vi "Test Process Wait For Lifecycle State After Clearing Throws Error.vi"(8 "error in (no error)":errorcluster, 11 "Process Test In":refnum<class "Process Dev Test.lvclass">) -> (0 "error out":errorcluster, 3 "Process Test Out":refnum<class "Process Dev Test.lvclass">)   [LabVIEW 2020, in "Process Dev Test.lvclass"]
uses:
  Process Dev Test.lvclass
  C:/Program Files (x86)/National Instruments/LabVIEW 2020/vi.lib/Astemes/LUnit/Test Case.lvclass
  source/Framework/Process/Public/Lifecycle/Lifecycle State.ctl
  <vilib>/Astemes/LUnit/Test Case.lvclass/Test Case.ctl
  <vilib>/Astemes/LUnit/LUnit Assertion Result.lvclass/LUnit Assertion Result.ctl
  <vilib>/Astemes/LUnit/LUnit Test Case Result.lvclass/LUnit Test Case Result.ctl
  <vilib>/Astemes/LUnit/LUnit Method Result.lvclass/LUnit Method Result.ctl
  <vilib>/Astemes/LUnit/Palette/Fail.vi
  <vilib>/Astemes/LUnit/Palette/Pass.vi
  <vilib>/Astemes/LUnit/Set Assertion Type.vi
  <vilib>/Astemes/LUnit/Add test result.vi
  <vilib>/Astemes/LUnit/LUnit Write Passed.vi
  <vilib>/Astemes/LUnit/LUnit Write Message.vi
  <vilib>/Astemes/LUnit/LUnit Write Description.vi
  <vilib>/Astemes/LUnit/LUnit Write Assertion Type.vi
  <vilib>/Astemes/LUnit/LUnit Record Assertion Result.vi
  <vilib>/Astemes/LUnit/LUnit Aggregate Assertion Results.vi
  <vilib>/Astemes/LUnit/Assertion Result/LUnit Read Status.vi
  <vilib>/Astemes/LUnit/LUnit Read Message.vi
  <vilib>/Astemes/LUnit/LUnit Read Description.vi
  <vilib>/Astemes/LUnit/Method Result/LUnit Merge Status.vi
  <vilib>/Astemes/LUnit/LUnit Concatenate result strings.vi
  <vilib>/Astemes/LUnit/LUnit Assertion Result.lvclass
  source/Framework/Process/Process.lvclass
  <vilib>/Astemes/LUnit/Test Case.lvclass
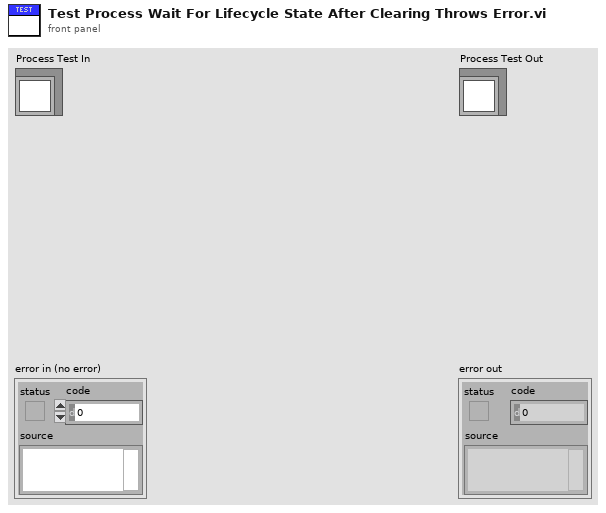
[diagram p1: front panel]
types:
  T1 = typedef "Process.lvclass/Lifecycle State.ctl" = enum16{"Uninitialized", "Initialized", "Started", "Running", "Stopped", "Finished"}
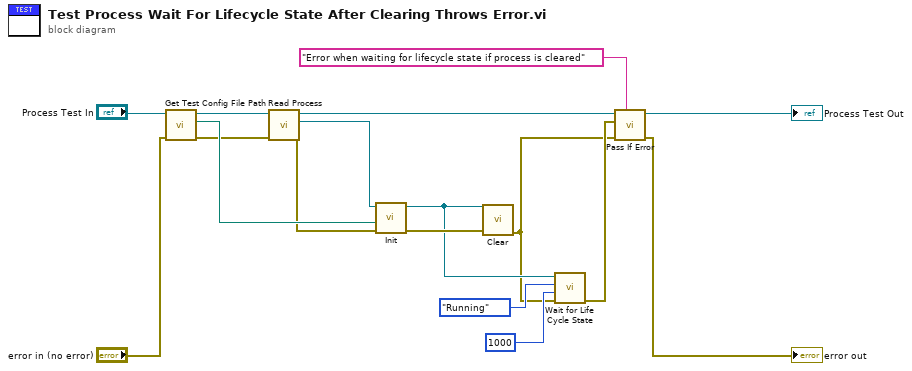
[diagram p0: block diagram]
diagram:
  n1 = call "Get Test Config File Path.vi"("error in (no error)"="error in (no error)", "Process Test In"="Process Test In") -> ("error out"=w10:errorcluster, "Test config path"=w13:path, "Process Test Out"=w15:refnum<class "Process Dev Test.lvclass">)  [unwired: 7 in]
  n2 = call "Read Process.vi"("error in (no error)"=w10, "Process Test in"=w15) -> ("error out"=w11:errorcluster, "Process.lvclass"=w12:refnum<class "Process.lvclass">, "Process Test out"=w6:refnum<class "Process Dev Test.lvclass">)  [unwired: 7 in]
  n3 = call-dynamic "Init.vi"("error in (no error)"=w11, "Config File Path"=w13, "Process In"=w12) -> ("error out"=w16:errorcluster, "Process Out"=w9:refnum<class "Process.lvclass">)  [unwired: 7 in]
  n4 = call-dynamic "Clear.vi"("error in (no error)"=w16, "Process In"=w9) -> ("error out"=w1:errorcluster)  [unwired: 9 in]
  n5 = call "Wait for Life Cycle State.vi"("error in (no error)"=w1, "timeout in ms (-1)"=1000, "Lifecycle State"=Lifecycle_State."Running", "Process In"=w9) -> ("error out"=w8:errorcluster)  [unwired: 5 in, 2 out]
  n6 = call <vilib>:"Pass If Error.vi"("Description"="Error when waiting for lifecycle state if process is cleared", "error in (no error)"=w1, "Assert error"=w8, "LUnit Test Case In"=w6) -> ("error out"=→"error out":errorcluster, "LUnit Test Case Out"=→"Process Test Out":refnum<class "Process Dev Test.lvclass">)  [unwired: 6 in]
